vi "S2C_FORNAX_Proc_UpdateParameters.vi"(8 "Error In":errorcluster, 9 "Row":i32, 10 "CtlRef":refnum<vi>, 11 "ItemTag":string) -> (0 "Error Out":errorcluster)   [LabVIEW 2015]
doc: "Finds the Int value for a selected Fornax command type."
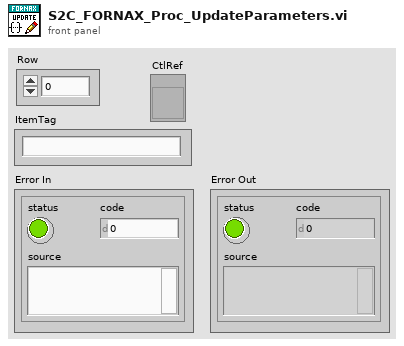
[diagram p1: front panel]
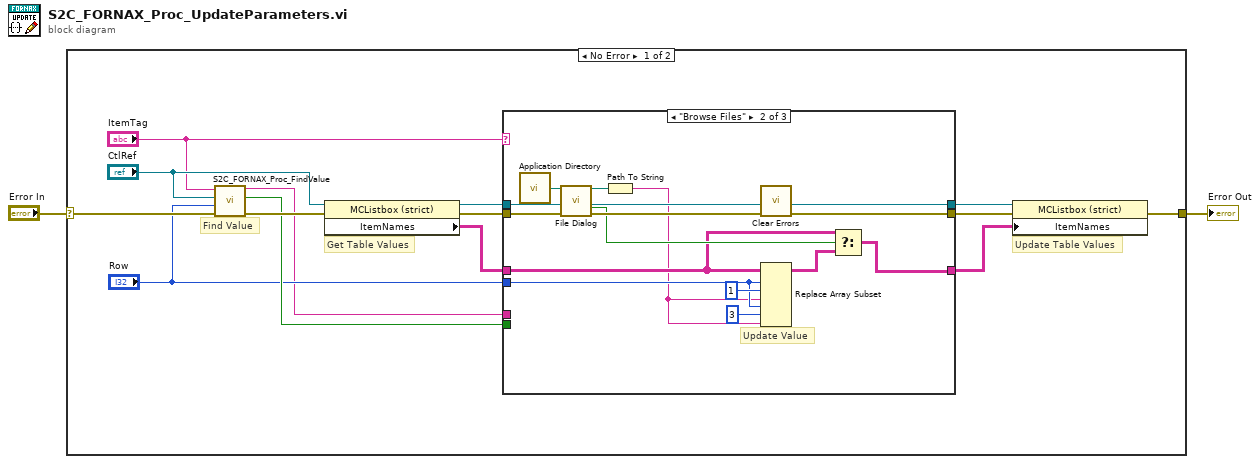
[diagram p0: block diagram]
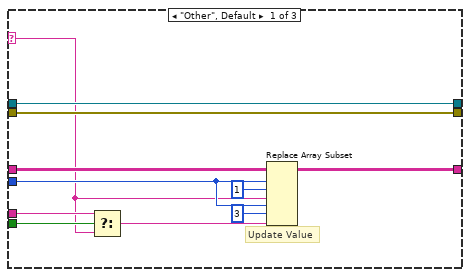
[diagram p2: hidden frame]
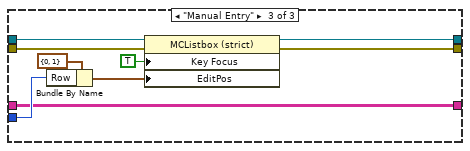
[diagram p3: hidden frame]
diagram:
  n1 = case shown="No Error" "Error In" {
    selector: "Error In" -> [w16 w51]
    tunnel: [w5 w51] -> w1
    frame No Error {
      # "Get Table Values"
      # "Update Table Values"
      # "Find Value"
      n2 = call "S2C_FORNAX_Proc_FindValue.vi"("Error In"=w16, "Row"="Row", "CtlRef"="CtlRef", "ItemTag"="ItemTag") -> ("Error Out"=w13:errorcluster, "Found?"=w12:bool, "Value_Int"=w10:string)  [unwired: 5 in]
      n3 = property on="Property Node" class="MCListbox (strict)"(reference="CtlRef", error in=w13) -> (reference out=w4:refnum<vi>, error out=w8:errorcluster, "ItemNames"=w14:string[][])
      n4 = case shown="\"Browse Files\"" "ItemTag" {
        selector: "ItemTag" -> [w17 _ _]
        tunnel: [w24 w33 w42] -> w15
        tunnel: w14 -> [w19 w35 w42]
        tunnel: w12 -> [w23 _ _]
        tunnel: "Row" -> [w18 w31 w43]
        tunnel: w10 -> [w22 _ _]
        tunnel: w8 -> [w21 w39 w45]
        tunnel: [w21 w28 w48] -> w7
        tunnel: w4 -> [w20 w32 w44]
        tunnel: [w20 w32 w49] -> w3
        frame "Other", Default {
          # "Update Value"
          n5 = Select(t=w22, s=w23, f=w17) -> (s? t:f=w27:string)
          n6 = Replace Array Subset(array=w19, new element #1=w17, index (row) #1=w18, index (col) #1=1 ("disabled index (col)"), new element #2=w27, index (row) #2=w18, index (col) #2=3 ("disabled index (col)")) -> (w24:string[][])
        }
        frame "Browse Files" {
          # "Update Value"
          n7 = call <vilib>:"Application Directory.vi"() -> ("Application Directory"=w40:path)
          n8 = call "File Dialog"("start path"=w40, "error in"=w39) -> ("selected path"=w38:path, "cancelled"=w36:bool, "error out"=w37:errorcluster)  [unwired: 10 in, 1 out]
          n9 = Path To String(path=w38) -> (string=w29:string)
          n10 = call <vilib>:"Clear Errors.vi"("error in (no error)"=w37) -> ("error out"=w28:errorcluster)  [unwired: 5 in, 1 out]
          n11 = Replace Array Subset(array=w35, new element #1=w29, index (row) #1=w31, index (col) #1=1 ("disabled index (col)"), new element #2=w29, index (row) #2=w31, index (col) #2=3 ("disabled index (col)")) -> (w34:string[][])
          n12 = Select(t=w35, s=w36, f=w34) -> (s? t:f=w33:string[][])
        }
        frame "Manual Entry" {
          n13 = Bundle By Name(cluster=cluster{"Row":i32, "Column":i32} {"Row"=0, "Column"=1} ("Edit Position"), "Row"=w43) -> (w47:cluster{"Row":i32, "Column":i32})
          n14 = property on="Property Node" class="MCListbox (strict)"(reference=w44, error in=w45, "Key Focus"=TRUE, "EditPos"=w47) -> (reference out=w49:refnum<vi>, error out=w48:errorcluster)
        }
      }
      n15 = property on="Property Node" class="MCListbox (strict)"(reference=w3, error in=w7, "ItemNames"=w15) -> (error out=w5:errorcluster)  [unwired: 1 out]
    }
    frame Error {
    }
  }
  "Error Out" <- w1
